vi "PPS_USE_ONLY_ON_FPGA_ITSELF.vi"() -> ()   [LabVIEW 2015]
panel:
  out "Timekeepr Lock":bool
  out "Pulse Per Sec":bool
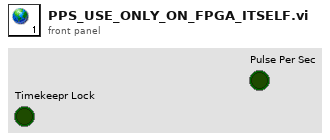
[diagram p1: front panel]
diagram:
